vi "Process.vi"(11 "Actor":refnum<class "Metronome Actor.lvclass">) -> ()   [LabVIEW 2015, in "Metronome Actor.lvclass"]
uses:
  Metronome Actor.lvclass
  Metronome Actor.lvclass/Metronome Actor.ctl
  Base Actor/Actor/Front Panel State.ctl
  Messaging/Message/Message.lvclass/Message.ctl
  Messaging/Message/Message.lvclass
  Utility/Utility.lvlib
  Base Actor/Actor/Actor.lvclass
panel:
  out "Metronome Name":string
  in  "Set Period [ms]":i32
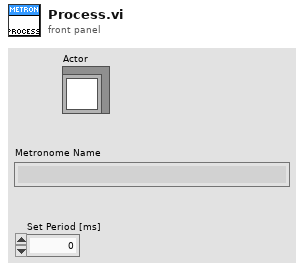
[diagram p1: front panel]
types:
  T1 = typedef "Actor.lvclass/Front Panel State.ctl" = enum32{"Invalid", "Standard", "Closed", "Hidden", "Minimized", "Maximized"}
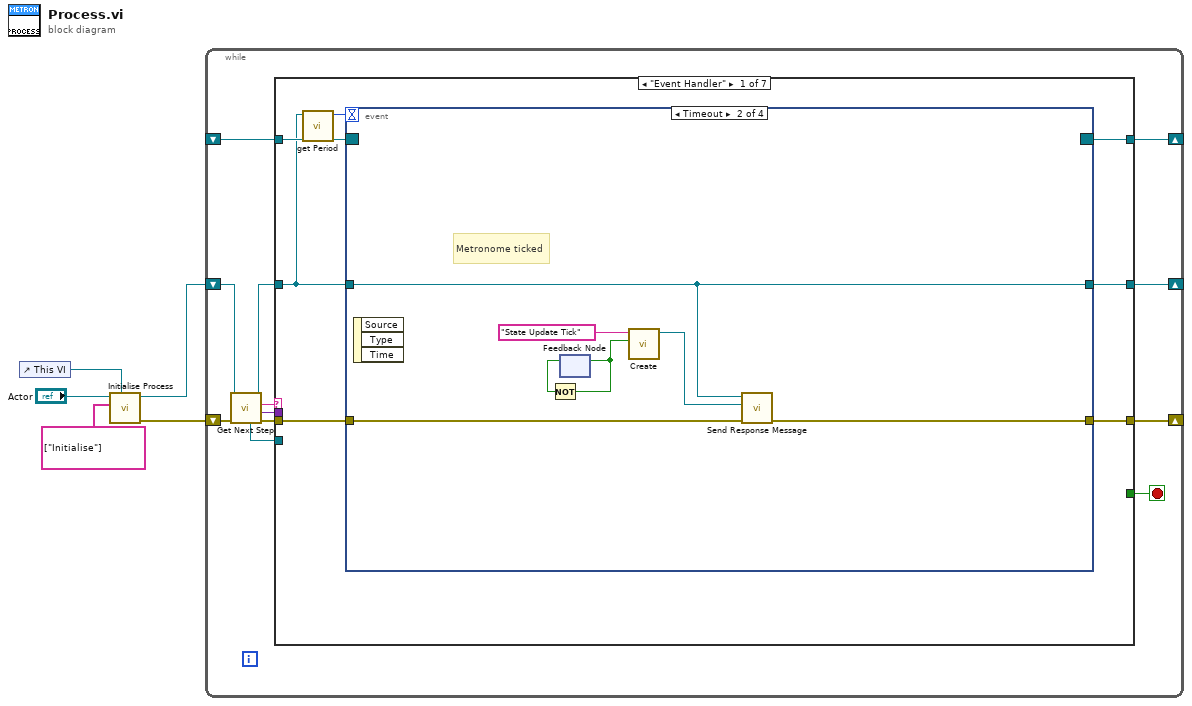
[diagram p0: block diagram]
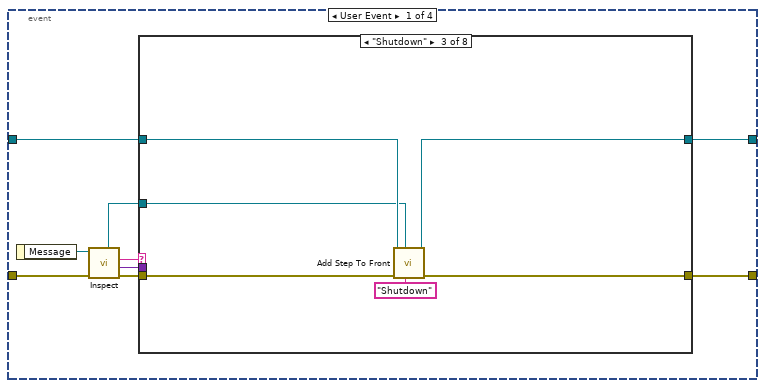
[diagram p2: hidden frame]
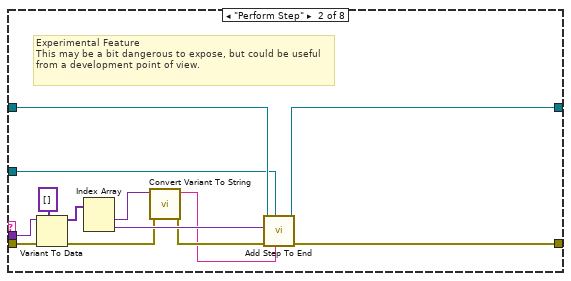
[diagram p4: hidden frame]
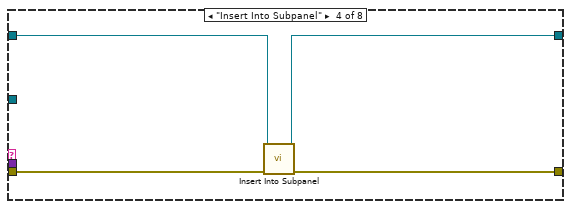
[diagram p5: hidden frame]
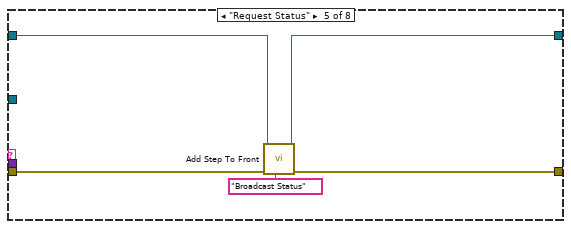
[diagram p6: hidden frame]
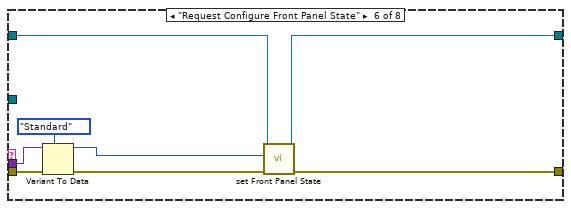
[diagram p7: hidden frame]
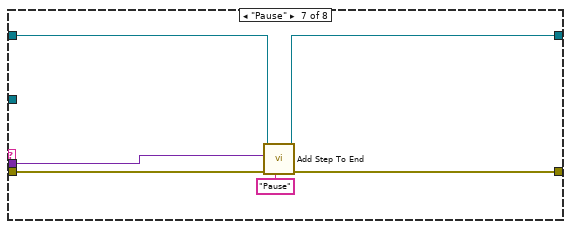
[diagram p8: hidden frame]
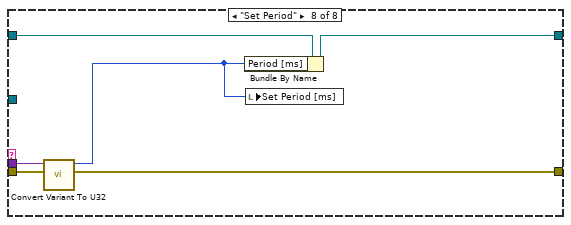
[diagram p9: hidden frame]
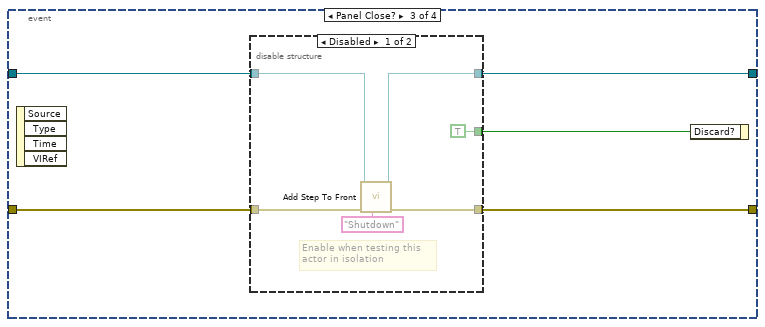
[diagram p10: hidden frame]
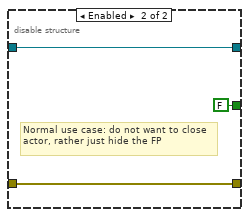
[diagram p11: hidden frame]
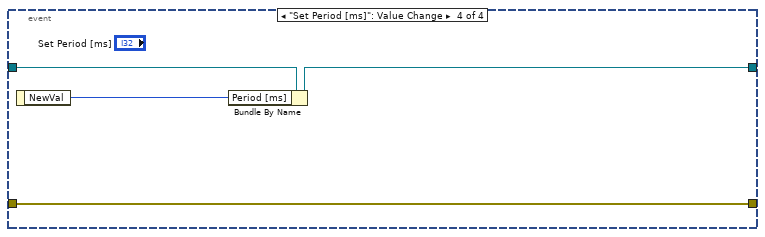
[diagram p12: hidden frame]
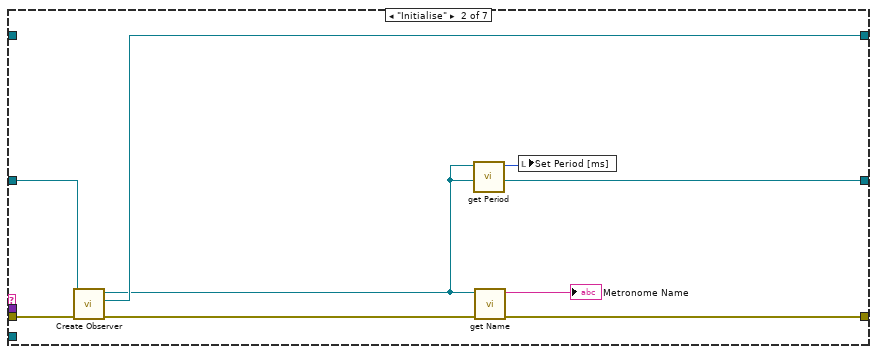
[diagram p13: hidden frame]
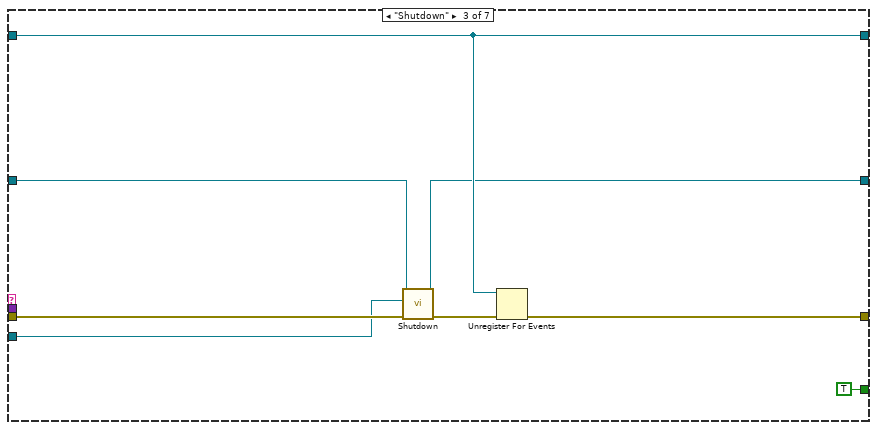
[diagram p14: hidden frame]
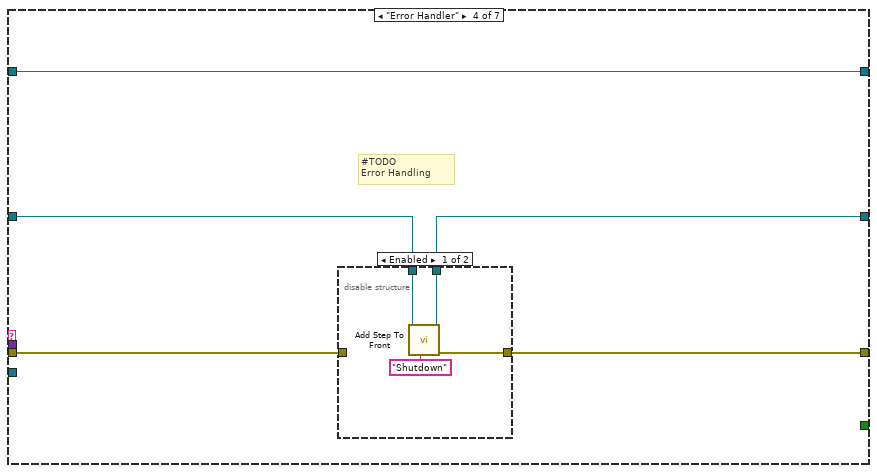
[diagram p15: hidden frame]
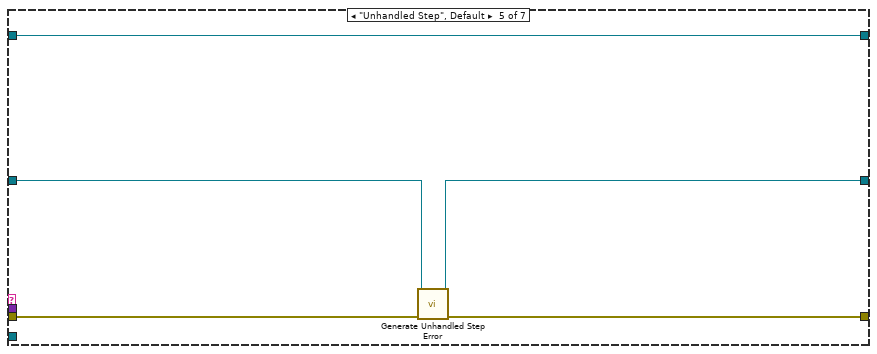
[diagram p17: hidden frame]
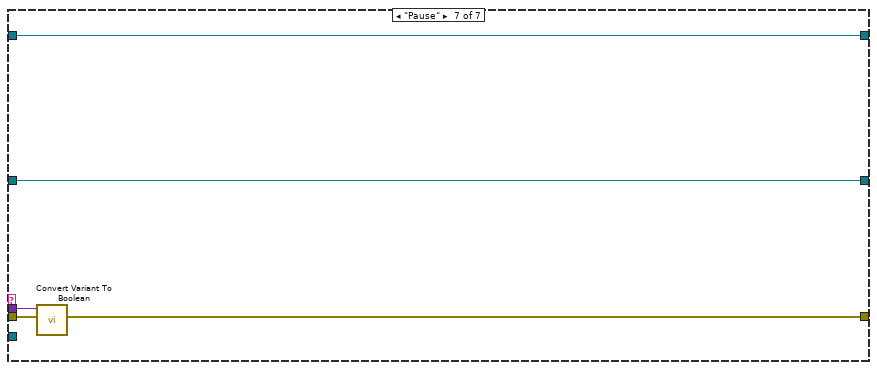
[diagram p19: hidden frame]
diagram:
  n1 = control-ref of="This VI"() -> (w1:refnum<vi>)
  n2 = call-dynamic "Initialise Process.vi"("Process"=w1, "Steps (Initialise)"=string[] ["Initialise"] ("Steps"), "Actor in"="Actor") -> ("error out"=w2:errorcluster, "Actor out"=w4:refnum<class "Metronome Actor.lvclass">)  [unwired: 7 in]
  n3 = while {
    shift-right: [w16] -> _
    shift-left: w4 -> [w15]
    shift-right: [w11] -> _
    shift-left: _ -> [w10]
    shift-right: [w8] -> _
    shift-left: w2 -> [w7]
    stop <- w17 stop-if-true
    n4 = call-dynamic "Get Next Step.vi"("error in (no error)"=w7, "Actor in"=w15) -> ("error out"=w9:errorcluster, "Parameter"=w12:variant, "Step"=w13:string, "Actor out"=w14:refnum<class "Metronome Actor.lvclass">, "Reply Channel"=w6:refnum<notifier>)  [unwired: 5 in]
    n5 = case shown="\"Event Handler\"" w13 {
      tunnel: [_ _ TRUE _ _ _ _] -> w17
      tunnel: w14 -> [w19 w116 w118 w127 w138 w141 w144]
      tunnel: [w24 w110 w121 w126 w137 w141 w144] -> w16
      tunnel: w12 -> [_ _ _ _ _ _ w146]
      tunnel: [w22 w115 w123 w129 w139 w142 w147] -> w11
      tunnel: w10 -> [w23 _ w123 w129 w139 w142 w147]
      tunnel: w9 -> [w21 w114 w120 w125 w136 w140 w145]
      tunnel: [w20 w113 w122 w128 w135 w140 w143] -> w8
      tunnel: w6 -> [_ _ w117 _ _ _ _]
      frame "Event Handler" {
        n6 = call "get Period.vi"("Metronome Actor in"=w19) -> ("Period [ms]"=w18:i32)  [unwired: 8 in]
        n7 = event shown="[1] Timeout" {
          selector: w23 -> [_ _ _ _]
          dyn-events: [_ _ _ _] -> w22
          timeout: w18 -> [_ _ _ _]
          tunnel: w19 -> [w33 w85 w91 w108]
          tunnel: [w32 w85 w92 w107] -> w24
          tunnel: w21 -> [w30 w88 w95 w105]
          tunnel: [w31 w87 w94 w105] -> w20
          event User Event {
            n8 = event-data() -> ("Message"=w29:refnum<class "Message.lvclass">)  [unwired: 1 in]
            n9 = call "Inspect.vi"("error in (no error)"=w30, "Message in"=w29) -> ("error out"=w26:errorcluster, "Data"=w27:variant, "Name"=w28:string, "Reply Channel"=w25:refnum<notifier>)  [unwired: 5 in, 1 out]
            n10 = case shown="\"Shutdown\"" w28 {
              tunnel: w33 -> [w35 w48 w54 w58 w63 w71 w77 w82]
              tunnel: [w35 w47 w53 w57 w62 w70 w76 w81] -> w32
              tunnel: w26 -> [w34 w45 w51 w56 w60 w68 w73 w80]
              tunnel: [w34 w46 w50 w55 w59 w69 w74 w79] -> w31
              tunnel: w27 -> [_ w37 _ _ _ w65 w72 w83]
              tunnel: w25 -> [_ w36 w49 _ _ _ _ _]
              frame Default {
              }
              frame "Perform Step" {
                # "Experimental Feature\nThis may be a bit dangerous to expose, but could be useful from a development point of view."
                n11 = Variant To Data(error in=w45, type=variant[] [], Variant=w37) -> (data=w43:variant[], error out=w40:errorcluster)
                n12 = Index Array(array=w43) -> (element #1=w41:variant, element #2=w42:variant)  [unwired: 2 in]
                n13 = call "Convert Variant To String.vi"("error in (no error)"=w40, "Variant"=w41) -> ("error out"=w39:errorcluster, "String"=w38:string)  [unwired: 8 in]
                n14 = call-dynamic "Add Step To End.vi"("Step Name"=w38, "Reply Channel"=w36, "error in (no error)"=w39, "Parameter"=w42, "Actor in"=w48) -> ("error out"=w46:errorcluster, "Actor out"=w47:refnum<class "Metronome Actor.lvclass">)  [unwired: 5 in]
              }
              frame "Shutdown" {
                n15 = call-dynamic "Add Step To Front.vi"("Step Name"="Shutdown", "Reply Channel"=w49, "error in (no error)"=w51, "Actor in"=w54) -> ("error out"=w50:errorcluster, "Actor out"=w53:refnum<class "Metronome Actor.lvclass">)  [unwired: 6 in]
              }
              frame "Insert Into Subpanel" {
                n16 = call-dynamic "Insert Into Subpanel.vi"("error in (no error)"=w56, "Actor in"=w58) -> ("error out"=w55:errorcluster, "Actor out"=w57:refnum<class "Metronome Actor.lvclass">)  [unwired: 8 in]
              }
              frame "Request Status" {
                n17 = call-dynamic "Add Step To Front.vi"("Step Name"="Broadcast Status", "error in (no error)"=w60, "Actor in"=w63) -> ("error out"=w59:errorcluster, "Actor out"=w62:refnum<class "Metronome Actor.lvclass">)  [unwired: 7 in]
              }
              frame "Request Configure Front Panel State" {
                n18 = Variant To Data(error in=w68, type=Front_Panel_State."Standard" ("Front Panel State"), Variant=w65) -> (data=w64:T1, error out=w67:errorcluster)
                n19 = call-dynamic "set Front Panel State.vi"("error in (no error)"=w67, "Front Panel State"=w64, "Actor in"=w71) -> ("error out"=w69:errorcluster, "Actor out"=w70:refnum<class "Metronome Actor.lvclass">)  [unwired: 7 in]
              }
              frame "Pause" {
                n20 = call-dynamic "Add Step To End.vi"("Step Name"="Pause", "error in (no error)"=w73, "Parameter"=w72, "Actor in"=w77) -> ("error out"=w74:errorcluster, "Actor out"=w76:refnum<class "Metronome Actor.lvclass">)  [unwired: 6 in]
              }
              frame "Set Period" {
                n21 = call "Convert Variant To U32.vi"("error in (no error)"=w80, "Variant"=w83) -> ("error out"=w79:errorcluster, "Numeric"=w78:u32)  [unwired: 8 in]
                n22 = Bundle By Name(cluster=w82, "Period [ms]"=w78) -> (w81:refnum<class "Metronome Actor.lvclass">)
                n23 = local write "Set Period [ms]"(w78) -> ()
              }
            }
          }
          event Timeout {
            # "Metronome ticked"
            n24 = event-data() -> ()  [unwired: 1 in, 3 out]
            n25 = feedback #1() -> (w90:bool)  [unwired: 1 in]
            n26 = Not(x=w90) -> (.not. x?=w86:bool)
            n27 = feedback-in #1(w86) -> ()
            n28 = call "Create.vi"("Data"=w86, "Name"="State Update Tick") -> ("Message out"=w89:refnum<class "Message.lvclass">)  [unwired: 8 in, 1 out]
            n29 = call-dynamic "Send Response Message.vi"("error in (no error)"=w88, "Message"=w89, "Actor in"=w85) -> ("error out"=w87:errorcluster)  [unwired: 8 in]
          }
          event Panel Close? {
            n30 = event-data() -> ()  [unwired: 1 in, 4 out]
            n31 = disable-structure shown="Disabled" {
              disable-tunnel: w95 -> [w100 w103]
              disable-tunnel: [w99 w103] -> w94
              disable-tunnel: w91 -> [w98 w104]
              disable-tunnel: [w97 w104] -> w92
              disable-tunnel: [TRUE ("Discard?") FALSE ("Discard?")] -> w93
              frame Disabled {
                # "Enable when testing this actor in isolation"
                n32 = call-dynamic "Add Step To Front.vi"("Step Name"="Shutdown", "error in (no error)"=w100, "Actor in"=w98) -> ("error out"=w99:errorcluster, "Actor out"=w97:refnum<class "Metronome Actor.lvclass">)  [unwired: 7 in]
              }
              frame Enabled {
                # "Normal use case: do not want to close actor, rather just hide the FP"
              }
            }
            n33 = event-data("Discard?"=w93) -> ()  [unwired: 1 in, 1 out]
          }
          event "Set Period [ms]": Value Change {
            n34 = event-data() -> ("NewVal"=w106:i32)  [unwired: 1 in]
            n35 = Bundle By Name(cluster=w108, "Period [ms]"=w106) -> (w107:refnum<class "Metronome Actor.lvclass">)
          }
        }
      }
      frame "Initialise" {
        n36 = call-dynamic "Create Observer.vi"("error in (no error)"=w114, "Actor in"=w116) -> ("error out"=w112:errorcluster, "Actor"=w115:refnum<event-registration>, "Actor out"=w110:refnum<class "Metronome Actor.lvclass">)  [unwired: 7 in]
        n37 = call "get Period.vi"("Metronome Actor in"=w110) -> ("Period [ms]"=w109:i32)  [unwired: 8 in]
        n38 = call-dynamic "get Name.vi"("error in (no error)"=w112, "Actor in"=w110) -> ("error out"=w113:errorcluster, "Name"=→"Metronome Name":string)  [unwired: 8 in]
        n39 = local write "Set Period [ms]"(w109) -> ()
      }
      frame "Shutdown" {
        n40 = call-dynamic "Shutdown.vi"("error in (no error)"=w120, "Reply Channel"=w117, "Actor in"=w118) -> ("error out"=w119:errorcluster, "Actor out"=w121:refnum<class "Metronome Actor.lvclass">)  [unwired: 7 in]
        n41 = Unregister For Events(event registration refnum=w123, error in=w119) -> (error out=w122:errorcluster)
      }
      frame "Error Handler" {
        # "#TODO\nError Handling"
        n42 = disable-structure shown="Enabled" {
          disable-tunnel: [w132 w134] -> w128
          disable-tunnel: w127 -> [w131 _]
          disable-tunnel: [w130 _] -> w126
          disable-tunnel: w125 -> [_ w134]
          frame Enabled {
            n43 = call-dynamic "Add Step To Front.vi"("Step Name"="Shutdown", "Actor in"=w131) -> ("error out"=w132:errorcluster, "Actor out"=w130:refnum<class "Metronome Actor.lvclass">)  [unwired: 8 in]
          }
          frame Disabled {
          }
        }
      }
      frame "Unhandled Step", Default {
        n44 = call-dynamic "Generate Unhandled Step Error.vi"("error in (no error)"=w136, "Actor in"=w138) -> ("error out"=w135:errorcluster, "Actor out"=w137:refnum<class "Metronome Actor.lvclass">)  [unwired: 8 in]
      }
      frame "-----------------------" {
        # "Separator"
      }
      frame "Pause" {
        n45 = call "Convert Variant To Boolean.vi"("error in (no error)"=w145, "Variant"=w146) -> ("error out"=w143:errorcluster)  [unwired: 8 in, 1 out]
      }
    }
  }
